vi "Add Line Feed to String.vi"(2 "String":string) -> (7 "String\\n":string)   [LabVIEW 2021, in "Strings.lvlib"]
doc: "Adds line feed to the string only if it is not empty"
uses:
  Strings.lvlib
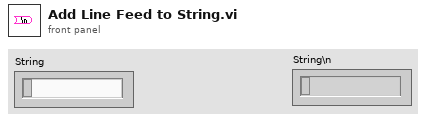
[diagram p1: front panel]
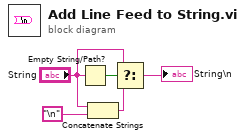
[diagram p0: block diagram]
diagram:
  n1 = Empty String/Path?(string/path="String") -> (empty?=w4:bool)
  n2 = Concatenate Strings("String", "\n") -> (w2:string)
  n3 = Select(t="String", s=w4, f=w2) -> (s? t:f=→"String\\n":string)
